vi "ESP8266 Blink LED.vi"(8 "Error In":errorcluster) -> (0 "Error Out":errorcluster)   [LabVIEW 2014]
uses:
  <vilib>/LabVIEW Universal Transcriptor/LabVIEW to Arduino Transcriptor/Transcriptors/System API/Serial println string.vi
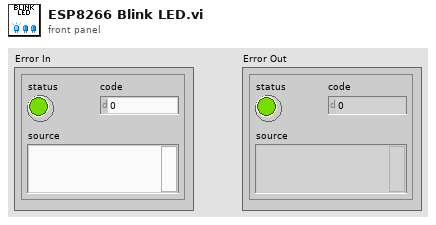
[diagram p1: front panel]
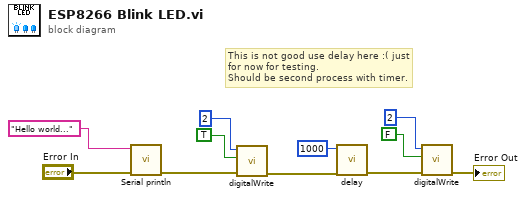
[diagram p0: block diagram]
diagram:
  # "This is not good use delay here :( just for now for testing.\nShould be second process with timer."
  n1 = call-poly <vilib>:"Serial println.vi"("Error In"="Error In", "string in"="Hello world...") -> ("Error Out"=w9:errorcluster)  [unwired: 9 in]
  n2 = call <vilib>:"digitalWrite.vi"("Error In"=w9, "value"=TRUE, "pin number"=2) -> ("Error Out"=w6:errorcluster)  [unwired: 8 in]
  n3 = call <vilib>:"delay.vi"("Error In"=w6, "time (ms)"=1000) -> ("Error Out"=w2:errorcluster)  [unwired: 9 in]
  n4 = call <vilib>:"digitalWrite.vi"("Error In"=w2, "value"=FALSE, "pin number"=2) -> ("Error Out"=→"Error Out":errorcluster)  [unwired: 8 in]
